vi "test_Read FXP Register Value.vi"(8 "error in (no error)":errorcluster, 11 "TestCase in":refnum<class "FPGA Register IO Tests.lvclass">) -> (0 "error out":errorcluster, 3 "TestCase out":refnum<class "FPGA Register IO Tests.lvclass">)   [LabVIEW 2020, in "FPGA Register IO Tests.lvclass"]
uses:
  FPGA Register IO Tests.lvclass
  FPGA Register IO Tests.lvclass/FPGA Register IO Tests.ctl
  APIs/FPGA Register IO/TypeDefs/FXP Configuration.ctl
  <vilib>/fxp/LVFixedPointRepBitsTypeDef.ctl
  <vilib>/fxp/LVFixedPointRepRangeTypeDef.ctl
  APIs/FPGA Register IO/Read Methods/Read Data Register/Instances/Read FXP.vi
  APIs/FPGA Register IO/SubVIs/FXP Raw to DBL.vi
  APIs/FPGA Register IO/Read Methods/Read Data Register/Instances/Read U16.vi
  APIs/FPGA Register IO/Read Methods/Read Data Register/Instances/Read U32.vi
  APIs/FPGA Register IO/Read Methods/Read Data Register/Instances/Read U64.vi
  APIs/FPGA Register IO/Read Methods/Read Data Register/Instances/Read U8.vi
  APIs/FPGA Register IO/Utilities/Find Register Offset.vi
  APIs/FPGA Register IO/SubVIs/Check Register Data Store.vi
  APIs/FPGA Register IO/Error Handling/Error 6001.vi
  APIs/FPGA Register IO/Error Handling/Error 6000.vi
  APIs/FPGA Register IO/Error Handling/Error 6002.vi
  APIs/FPGA Register IO/Error Handling/Error 6003.vi
  <vilib>/FPGAPlugInAG/Dynamic/niLvFpga_Close_Dynamic.vi
  <vilib>/rvi/interface/nirviCloseFPGA/nirviCloseFPGA.xnode
  <vilib>/addons/_JKI Toolkits/VI Tester/TestCase.llb/TestCase.lvclass
  APIs/FPGA Register IO/FPGA Register IO.lvlib
  C:/Program Files (x86)/National Instruments/LabVIEW 2020/vi.lib/addons/_JKI Toolkits/VI Tester/TestCase.llb/TestCase.lvclass
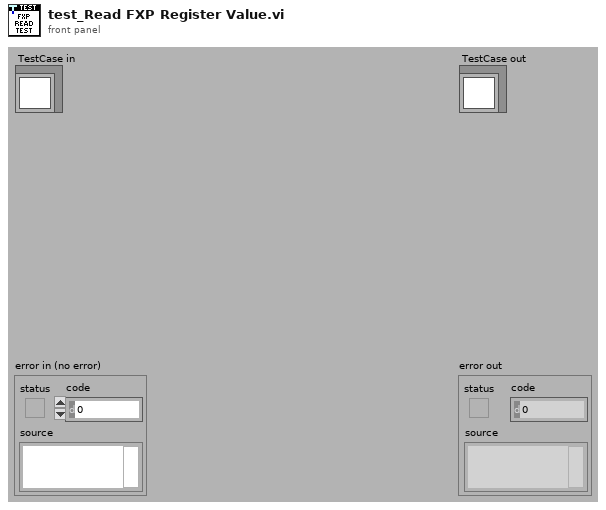
[diagram p1: front panel]
types:
  T1 = typedef "FPGA Register IO.lvlib/FXP Configuration.ctl" = cluster{"FXP Representation":T2, "FXP Range":T3}
  T2 = typedef "LVFixedPointRepBitsTypeDef.ctl" = cluster{"Signed":bool, "Word Length":u32, "Integer Word Length":i32}
  T3 = typedef "LVFixedPointRepRangeTypeDef.ctl" = cluster{"Range Min":dbl, "Range Max":dbl, "Delta":dbl}
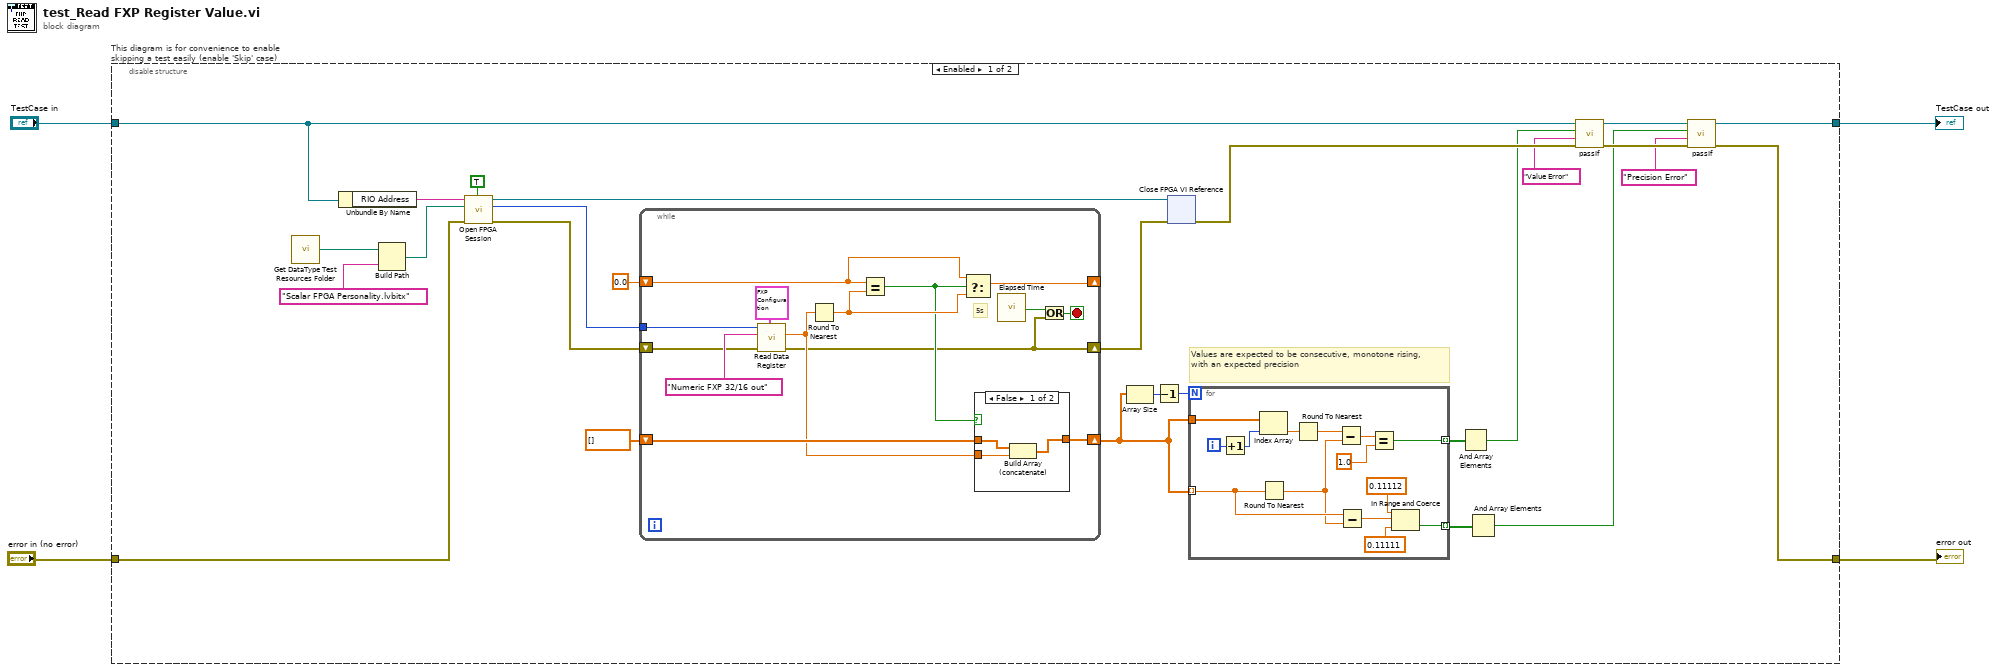
[diagram p0: block diagram]
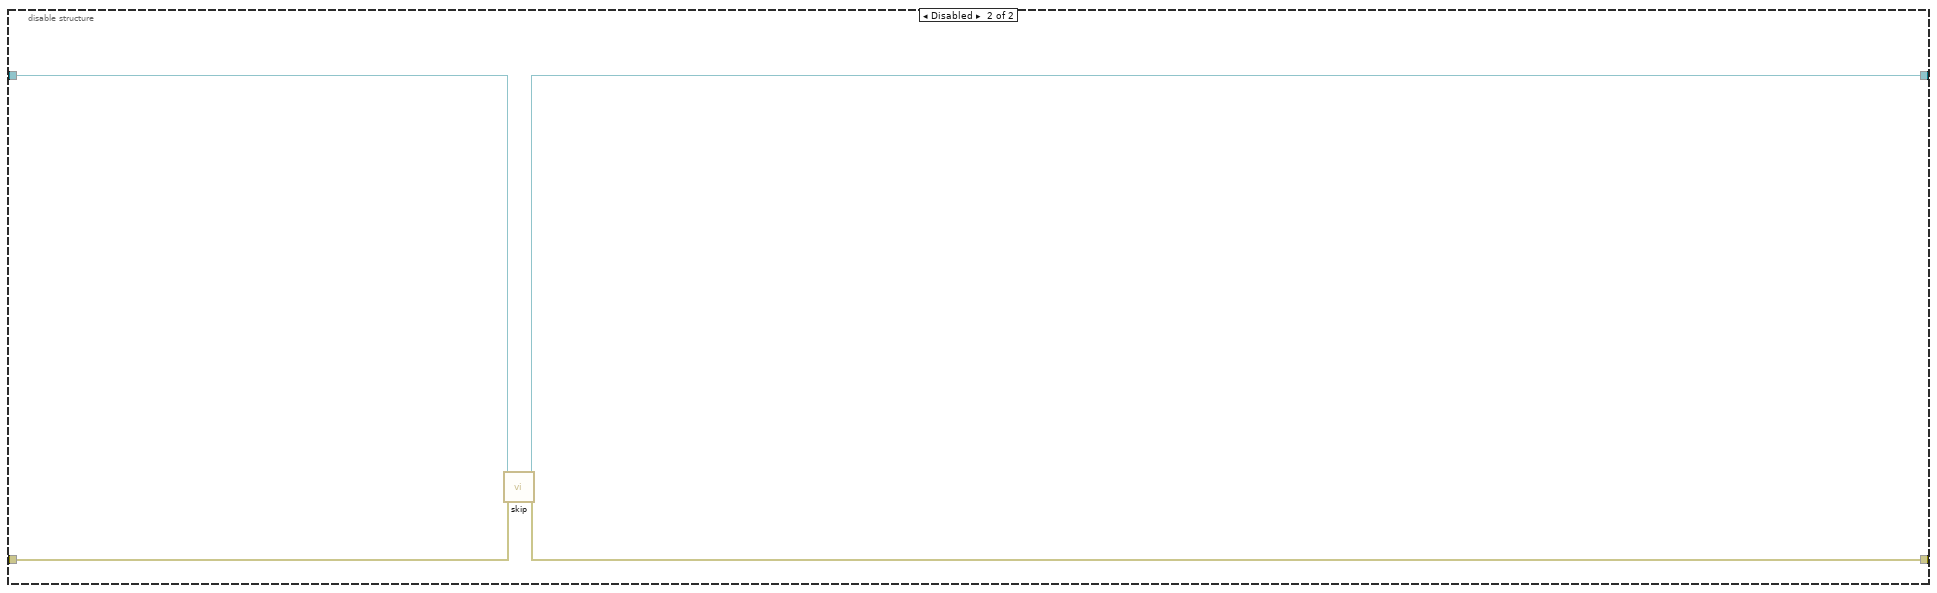
[diagram p3: hidden frame]
diagram:
  n1 = disable-structure "This diagram is for convenience to enable skipping a test easily (enable 'Skip' case)" shown="Enabled" {
    disable-tunnel: "TestCase in" -> [w16 w67]
    disable-tunnel: [w6 w65] -> w1
    disable-tunnel: [w7 w66] -> w3
    disable-tunnel: "error in (no error)" -> [w17 w64]
    frame Enabled {
      # "Values are expected to be consecutive, monotone rising, with an expected precision"
      n2 = call "Get DataType Test Resources Folder.vi"() -> ("path"=w14:path)
      n3 = Unbundle By Name(w16) -> ("RIO Address"=w19:string)
      n4 = Build Path(base path=w14, name or relative path="Scalar FPGA Personality.lvbitx") -> (appended path=w18:path)
      n5 = call "Open FPGA Session.vi"("run when loaded (T)"=TRUE ("Run When Loaded (T)"), "error in"=w17, "bitfile path"=w18, "device address"=w19) -> ("error out"=w25:errorcluster, "session out"=w24:u32, "bitfile reference out"=w23:refnum<k20>)  [unwired: 5 in]
      n6 = while {
        tunnel: w24 -> [w39]
        shift-right: [w32] -> w22
        shift-left: w25 -> [w37]
        shift-right: [w43] -> _
        shift-left: 0.0 ("DBL Value") -> [w45]
        shift-right: [w41] -> w26
        shift-left: dbl[] [] -> [w40]
        stop <- w34 stop-if-true
        # "5s"
        n7 = call-poly "Read Data Register.vi"("FXP Configuration"=T1 {"FXP Representation"={"Signed"=TRUE, "Word Length"=32, "Integer Word Length"=16}, "FXP Range"={"Range Min"=0.0, "Range Max"=0.0, "Delta"=1.52588e-05}}, "error in"=w37, "register name"="Numeric FXP 32/16 out" ("registerName"), "session in"=w39) -> ("error out"=w32:errorcluster, "DBL Value"=w36:dbl)  [unwired: 5 in, 1 out]
        n8 = Round To Nearest(number=w36) -> (nearest integer value=w44:dbl)
        n9 = Equal?(x=w45, y=w44) -> (x = y?=w42:bool)
        n10 = Select(t=w45, s=w42, f=w44) -> (s? t:f=w43:dbl)
        n11 = case shown="False" w42 {
          tunnel: w36 -> [w48 _]
          tunnel: [w47 w49] -> w41
          tunnel: w40 -> [w46 w49]
          frame False {
            n12 = Build Array (concatenate)(w46, w48) -> (w47:dbl[])
          }
          frame True {
          }
        }
        n13 = call "Elapsed Time"() -> ("Time has Elapsed"=w33:bool)  [unwired: 12 in, 7 out]
        n14 = Or(x=w33, y=w32) -> (x .or. y?=w34:bool)
      }
      n15 = Array Size(array=w26) -> (size(s)=w27:i32)
      n16 = Decrement(x=w27) -> (x-1=w28:i32)
      n17 = xnode "Close FPGA VI Reference"("FPGA VI Reference In"=w23, "error in"=w22) -> ("error out"=w15:errorcluster)
      n18 = for {
        N: w28 -> [_]
        tunnel: w26 -> [w58] mode=indexing
        tunnel: w26 -> [w63]
        tunnel: [w54] -> w29 mode=indexing
        tunnel: [w51] -> w30 mode=indexing
        i -> [w62]
        n19 = Increment(x=w62) -> (x+1=w61:i32)
        n20 = Index Array(array=w63, index=w61) -> (element=w60:dbl)
        n21 = Round To Nearest(number=w58) -> (nearest integer value=w57:dbl)
        n22 = Round To Nearest(number=w60) -> (nearest integer value=w59:dbl)
        n23 = Subtract(x=w59, y=w57) -> (x-y=w56:dbl)
        n24 = Subtract(x=w58, y=w57) -> (x-y=w50:dbl)
        n25 = Equal?(x=w56, y=1.0) -> (x = y?=w54:bool)
        n26 = In Range and Coerce(upper limit=0.11112, x=w50, lower limit=0.11111 ("upper limit")) -> (In Range?=w51:bool)  [unwired: 1 out]
      }
      n27 = And Array Elements(Boolean array=w29) -> (logical AND=w13:bool)
      n28 = And Array Elements(Boolean array=w30) -> (logical AND=w9:bool)
      n29 = call-dynamic "passIf.vi"("error in (no error)"=w15, "message (\"\")"="Value Error" ("message (\"\")"), "pass"=w13, "TestCase in"=w16) -> ("error out"=w11:errorcluster, "TestCase out"=w10:refnum<class "FPGA Register IO Tests.lvclass">)  [unwired: 6 in]
      n30 = call-dynamic "passIf.vi"("error in (no error)"=w11, "message (\"\")"="Precision Error" ("message (\"\")"), "pass"=w9, "TestCase in"=w10) -> ("error out"=w7:errorcluster, "TestCase out"=w6:refnum<class "FPGA Register IO Tests.lvclass">)  [unwired: 6 in]
    }
    frame Disabled {
      # "skip test result while test is under development"
      n31 = call <vilib>:"skip.vi"("error in (no error)"=w64, "TestCase in"=w67) -> ("error out"=w66:errorcluster, "TestCase out"=w65:refnum<class "FPGA Register IO Tests.lvclass">)  [unwired: 8 in]
    }
  }
  "error out" <- w3
  "TestCase out" <- w1
